vi "FinalLabview.vi"() -> ()   [LabVIEW 2021]
panel:
  out "ballcolor5":dbl
  out "ballcolor4":dbl
  out "ballcolor3":dbl
  out "ballcolor2":dbl
  out "ballcolor1":dbl
  out "DummyIndicator 5":dbl
  out "Ball Color":dbl
  out "DummyIndicator 3":dbl
  out "Ball Count":dbl
  out "Ball Color 5":string
  out "Ball Color 4":string
  out "Ball Color 3":string
  out "Ball Color 2":string
  out "Ball Color 1":string
  out "Y Coordinate 5":dbl
  out "X Coordinate 5":dbl
  out "Y Coordinate 4":dbl
  out "X Coordinate 4":dbl
  out "Y Coordinate 3":dbl
  out "X Coordinate 3":dbl
  out "Y Coordinate 2":dbl
  out "X Coordinate 2":dbl
  out "Robot Location":picture
  in  "Display History":bool
  in  "Size of Rectangle":i16
  out "Y Coordinate 1":dbl
  out "X Coordinate 1":dbl
  out "Y":dbl
  out "X":dbl
  in  "SendValue8":dbl
  in  "SendValue7":dbl
  in  "SendValue6":dbl
  in  "SendValue5":dbl
  in  "SendValue4":dbl
  in  "SendValue3":dbl
  in  "SendValue2":dbl
  in  "SendValue1":dbl
  in  "Send Button":bool
  in  "Stop Button":bool
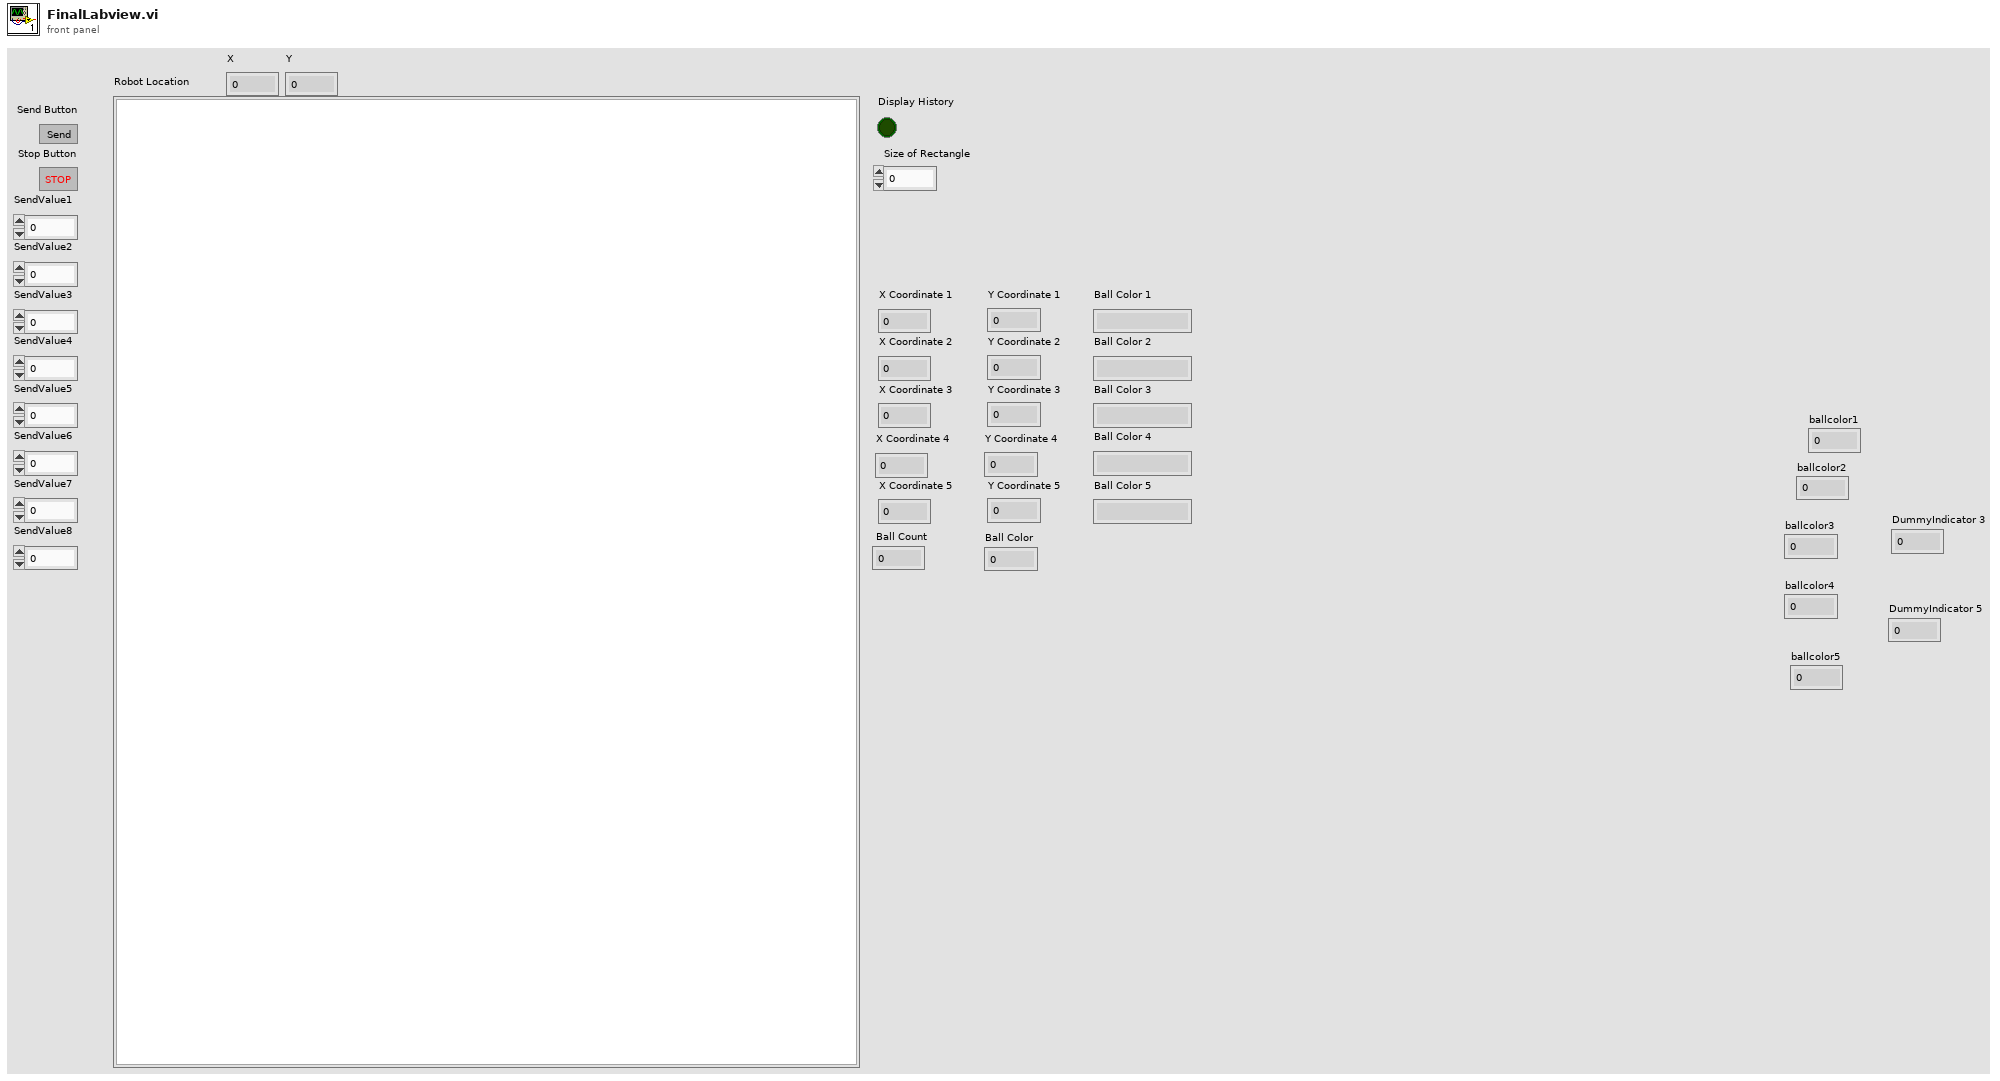
[diagram p1: front panel]
types:
  T1 = cluster{"Width":i16, "Style":enum32{"Solid", "Dash", "Dot", "DashDot", "DashDotDot"}}
  T2 = cluster{"left":i16, "top":i16, "right":i16, "bottom":i16}
  T3 = enum16{"Standard", "Buffered", "CRLF", "Immediate"}
  T4 = cluster{"Width":u16, "Style":enum32{"Solid", "Dash", "Dot", "DashDot", "DashDotDot"}}
  T5 = cluster{"default value 1":dbl, "default value 1":dbl}
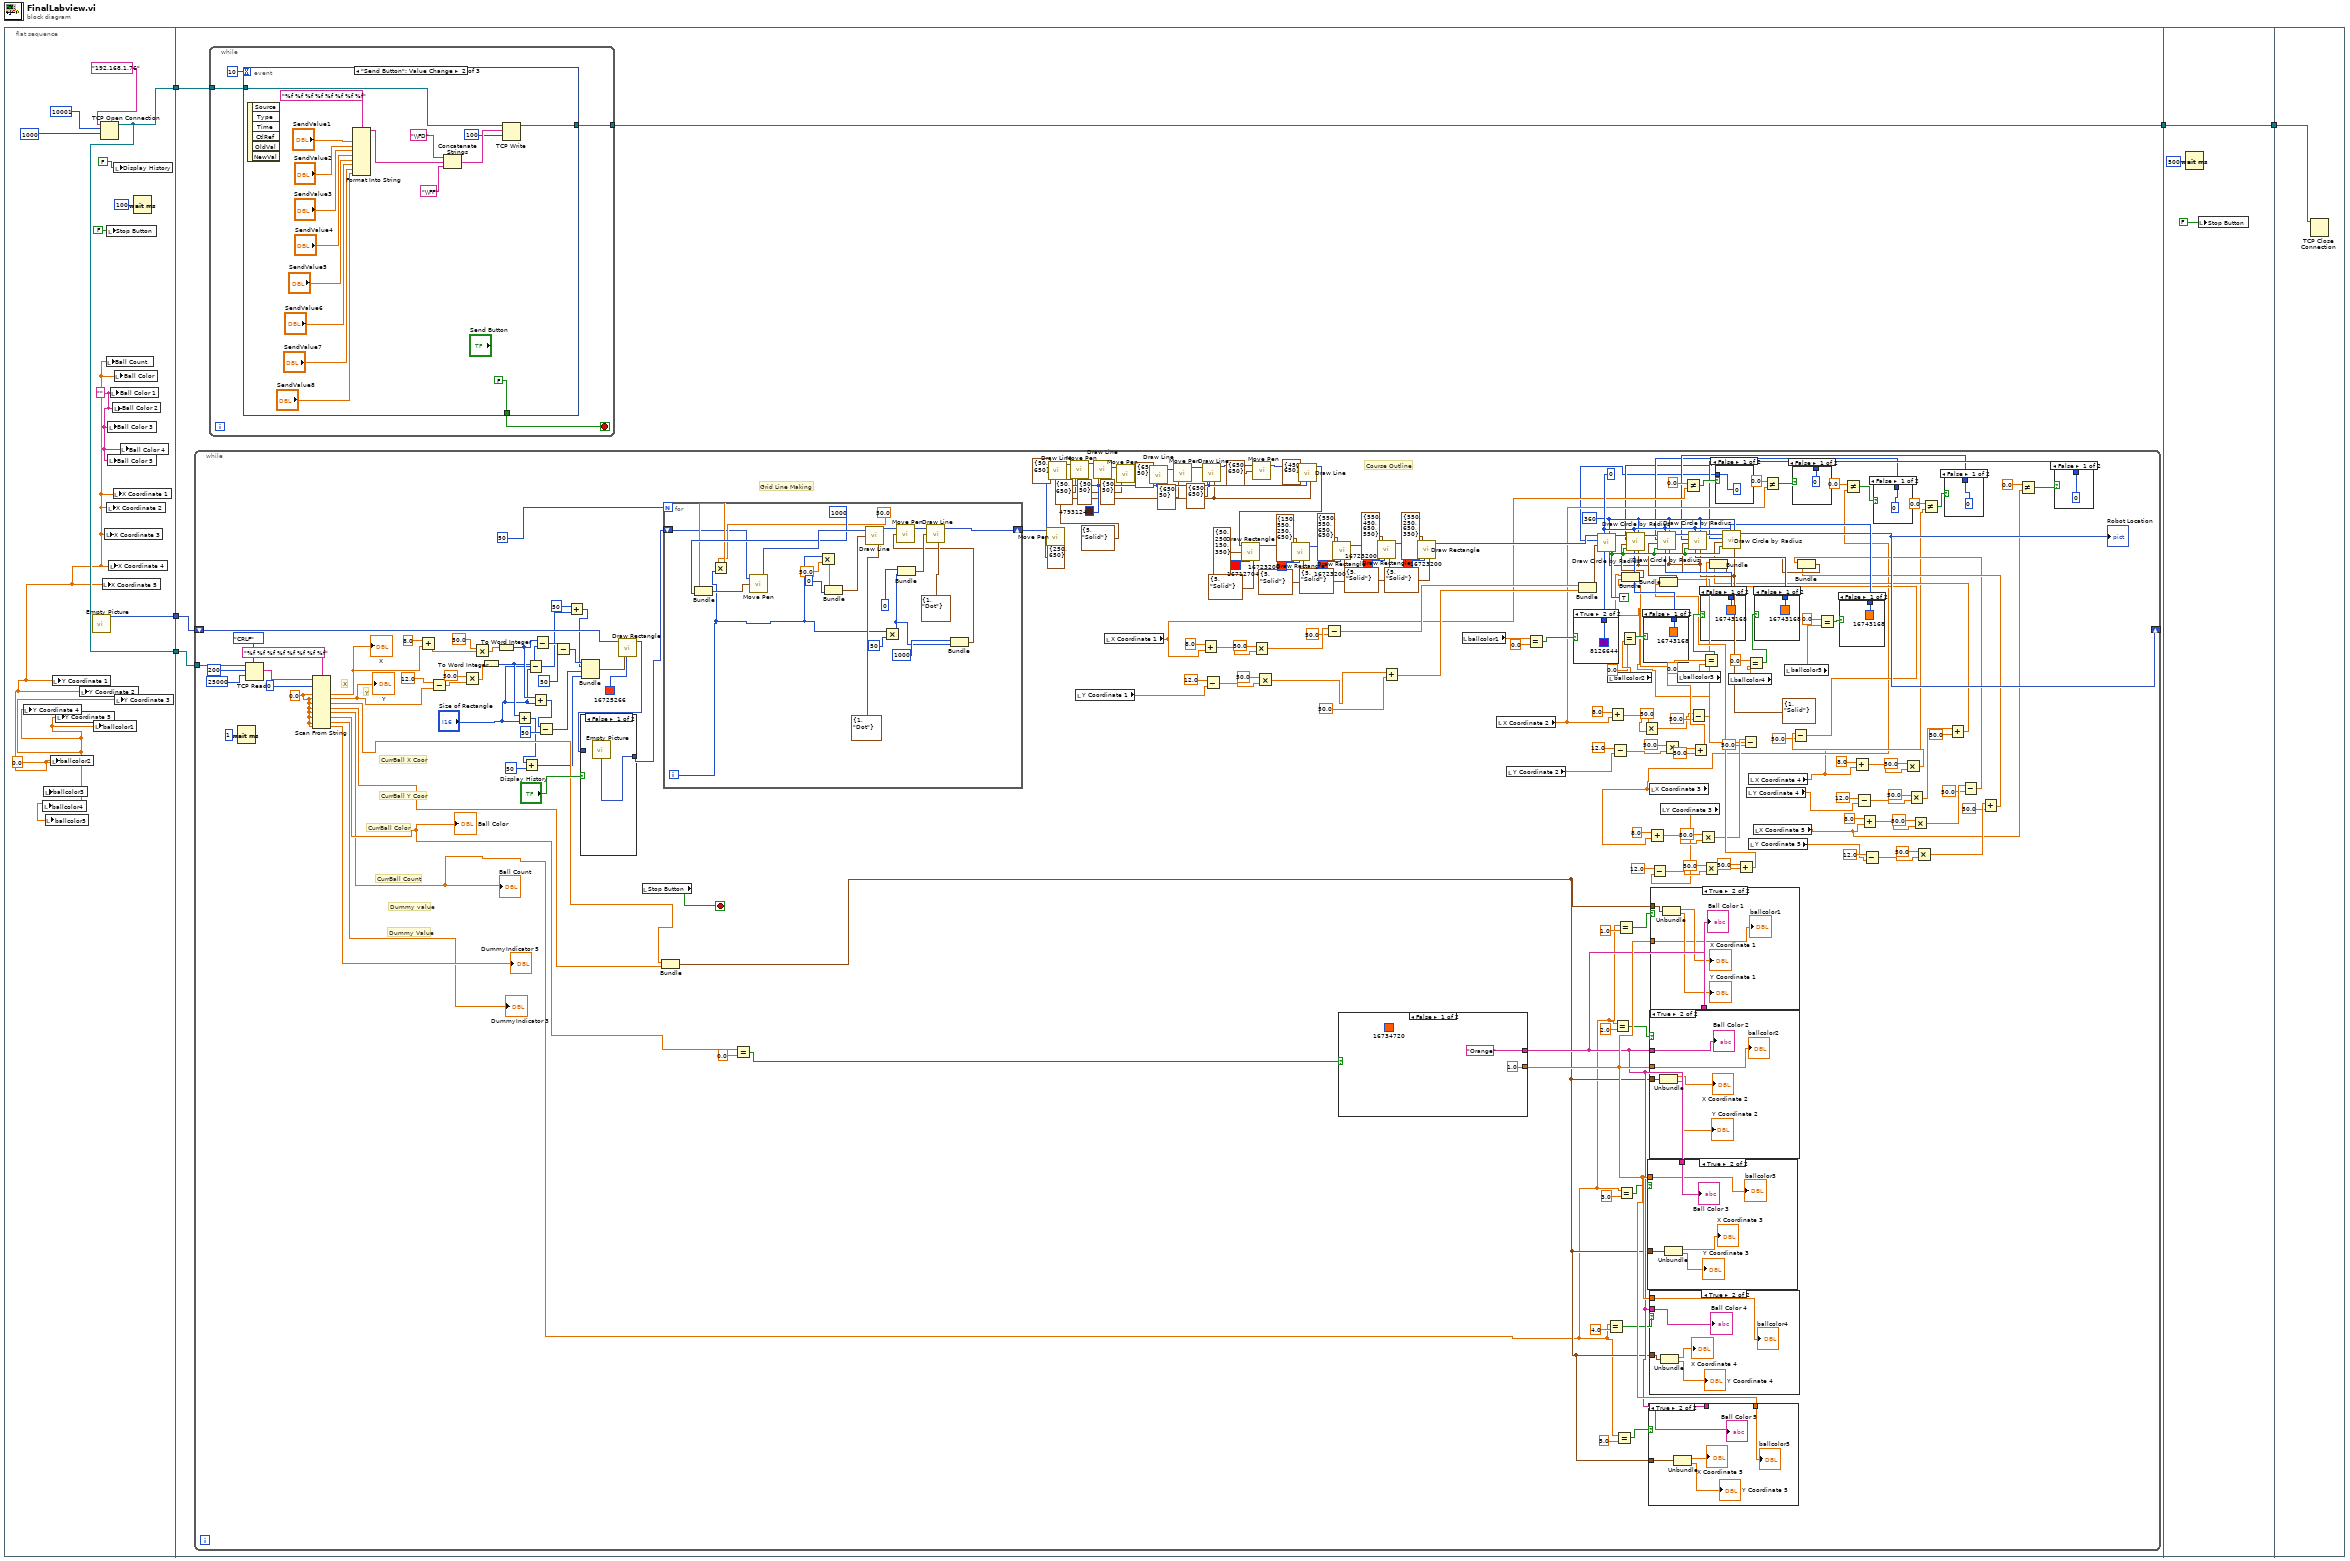
[diagram p0: block diagram]
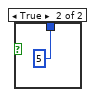
[diagram p2: hidden frame]
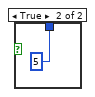
[diagram p3: hidden frame]
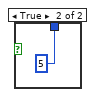
[diagram p4: hidden frame]
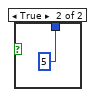
[diagram p5: hidden frame]
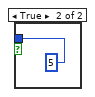
[diagram p6: hidden frame]
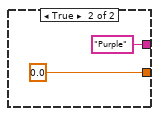
[diagram p12: hidden frame]
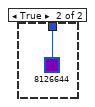
[diagram p13: hidden frame]
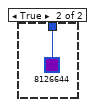
[diagram p14: hidden frame]
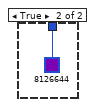
[diagram p15: hidden frame]
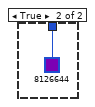
[diagram p16: hidden frame]
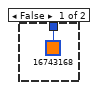
[diagram p17: hidden frame]
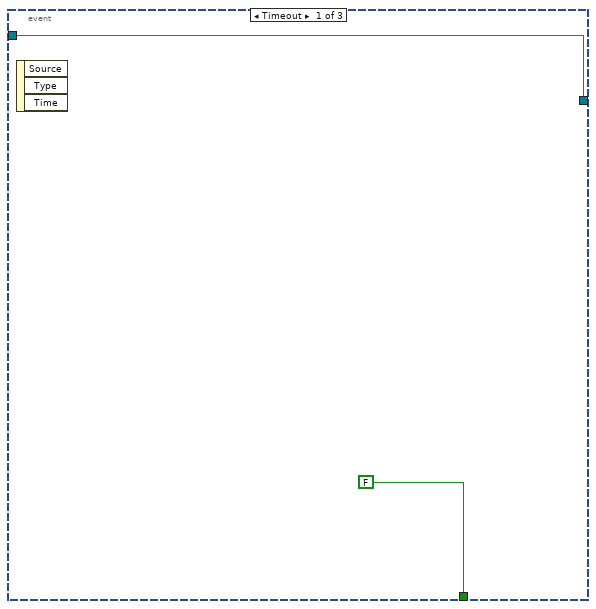
[diagram p19: hidden frame]
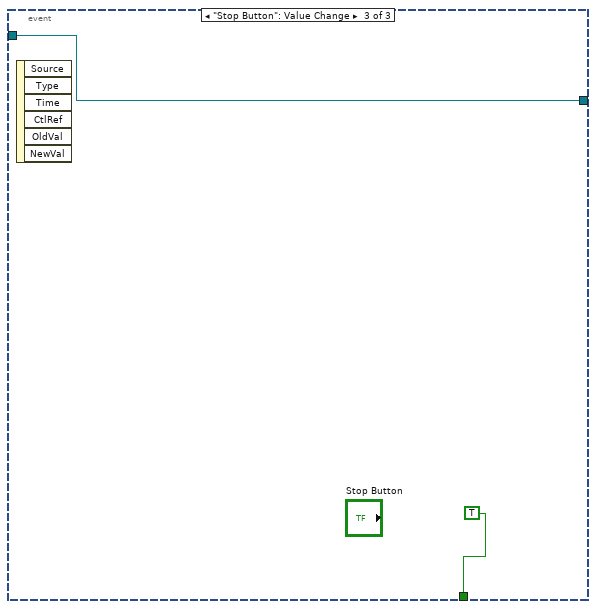
[diagram p20: hidden frame]
diagram:
  n1 = flat-sequence {
    tunnel: [w8] -> w5
    tunnel: [w10] -> w2
    tunnel: [w8] -> w1
    tunnel: w5 -> [w19]
    tunnel: [w18] -> w3
    tunnel: w2 -> [w16]
    tunnel: w1 -> [w17]
    tunnel: [w343] -> w4
    tunnel: w3 -> [w343]
    tunnel: w4 -> [w346]
    frame #0 {
      w6 = "" ("Ball Color 1")
      w7 = 0.0 ("ballcolor2")
      n2 = local write "Y Coordinate 4"(w7) -> ()
      n3 = local write "ballcolor4"(w7) -> ()
      n4 = local write "ballcolor3"(w7) -> ()
      n5 = local write "ballcolor5"(w7) -> ()
      n6 = local write "ballcolor2"(w7) -> ()
      n7 = local write "Y Coordinate 1"(w7) -> ()
      n8 = local write "Y Coordinate 5"(w7) -> ()
      n9 = local write "Y Coordinate 2"(w7) -> ()
      n10 = call "Empty Picture"() -> ("empty picture"=w10:picture)
      n11 = local write "ballcolor1"(w7) -> ()
      n12 = TCP Open Connection(address="192.168.1.76", remote port or service name=u16 10001, timeout ms (60000)=1000) -> (connection ID=w8:refnum<k5>)  [unwired: 2 in, 1 out]
      n13 = local write "X Coordinate 5"(w7) -> ()
      n14 = local write "X Coordinate 3"(w7) -> ()
      n15 = local write "Ball Count"(w7) -> ()
      n16 = local write "Stop Button"(FALSE) -> ()
      n17 = local write "X Coordinate 2"(w7) -> ()
      n18 = local write "Ball Color 3"(w6) -> ()
      n19 = local write "Ball Color 5"(w6) -> ()
      n20 = local write "X Coordinate 4"(w7) -> ()
      n21 = local write "Ball Color 1"(w6) -> ()
      n22 = local write "Ball Color 2"(w6) -> ()
      n23 = local write "X Coordinate 1"(w7) -> ()
      n24 = local write "Display History"(FALSE) -> ()
      n25 = local write "Ball Color"(w7) -> ()
      n26 = local write "Y Coordinate 3"(w7) -> ()
      n27 = local write "Ball Color 4"(w6) -> ()
      n28 = Wait (ms)(milliseconds to wait=u32 100) -> ()  [unwired: 1 out]
    }
    frame #1 {
      n29 = while {
        tunnel: w17 -> [w243]
        shift-right: [w126] -> _
        shift-left: w16 -> [w223]
        stop <- w220 stop-if-true
        w127 = T4 {"Width"=1, "Style"=enum."Solid"} ("pen")
        w152 = TRUE ("fill?(F)")
        w151 = i16 360 ("arc size(360)")
        w153 = i16 0 ("start angle(0)")
        w194 = T4 {"Width"=5, "Style"=enum."Solid"} ("pen")
        w195 = u32 4793124 ("color(black)")
        w175 = 0.0 ("default value 1")
        # "Dummy Value"
        # "CurrBall Count"
        # "Dummy value"
        # "CurrBall Color"
        # "CurrBall Y Coor"
        # "CurrBall X Coor"
        # "Y"
        # "X"
        # "Course Outline"
        # "Grid Line Making"
        n30 = Wait (ms)(milliseconds to wait=u32 1) -> ()  [unwired: 1 out]
        n31 = TCP Read(connection ID=w243, bytes to read=200, 7:T3."CRLF" ("mode (standard)"), 9:25000 ("timeout ms (25000)")) -> (data out=w239:string)  [unwired: 1 in, 2 out]
        n32 = Scan From String(format string="%f %f %f %f %f %f %f %f", input string=w239, initial scan location=u32 0, default 1=w175, default 2=w175, default 3=w175, default 4=w175, default 5=w175, default 6=w175, default 7=w175, default 8=w175) -> (output 1=w236:dbl, output 2=w174:dbl, output 3=w197:dbl, output 4=w172:dbl, output 5=w46:dbl, output 6=w169:dbl, output 7=→"DummyIndicator 3":dbl, output 8=→"DummyIndicator 5":dbl)  [unwired: 1 in, 3 out]
        "X" <- w236
        "Y" <- w174
        "Ball Count" <- w46
        "Ball Color" <- w169
        n33 = Add(x=8.0, y=w236) -> (x+y=w233:dbl)
        n34 = Subtract(x=12.0, y=w174) -> (x-y=w231:dbl)
        n35 = Multiply(x=50.0, y=w231) -> (x*y=w228:dbl)
        n36 = Multiply(x=50.0, y=w233) -> (x*y=w229:dbl)
        n37 = To Word Integer(number=w228) -> (16bit integer=w226:i16)
        n38 = To Word Integer(number=w229) -> (16bit integer=w227:i16)
        n39 = Add(x=w226, y="Size of Rectangle") -> (x+y=w44:i16)
        n40 = Add(x=w44, y=i16 50) -> (x+y=w45:i16)
        n41 = Subtract(x=w226, y="Size of Rectangle") -> (x-y=w42:i16)
        n42 = Add(x=w227, y="Size of Rectangle") -> (x+y=w164:i16)
        n43 = Subtract(x=w227, y="Size of Rectangle") -> (x-y=w161:i16)
        n44 = Subtract(x=w164, y=i16 50) -> (x-y=w163:i16)
        n45 = Subtract(x=w161, y=i16 50) -> (x-y=w162:i16)
        n46 = Add(x=i16 50, y=w42) -> (x+y=w40:i16)
        n47 = Bundle(w162, w40, w163, w45) -> (w222:cluster{i16, i16, i16, i16})  [unwired: 1 in]
        n48 = call <vilib>:"Draw Rectangle.vi"("picture"=w223, "rect"=w222, "color(black)"=u32 16725266) -> ("new picture"=w168:picture)  [unwired: 6 in]
        n49 = case shown="False" "Display History" {
          tunnel: w168 -> [_ w317]
          tunnel: [w316 w317] -> w167
          frame False {
            n50 = call "Empty Picture"() -> ("empty picture"=w316:picture)
          }
          frame True {
          }
        }
        n51 = local read "Stop Button"() -> (w220:bool)
        n52 = Bundle("default value 1"=w197, "default value 1"=w172) -> (w112:T5)  [unwired: 1 in]
        n53 = for {
          N: 50 -> [_]
          shift-right: [w310] -> w217
          shift-left: w167 -> [w294]
          i -> [w295]
          n54 = Multiply(x=50.0, y=w295) -> (x*y=w300:dbl)
          n55 = Bundle(w300, 1000) -> (w302:cluster{dbl, i32})  [unwired: 1 in]
          n56 = call <vilib>:"Move Pen.vi"("new position"=w302, "picture"=w294) -> ("new picture"=w306:picture)  [unwired: 3 in]
          n57 = Multiply(x=w295, y=50.0) -> (x*y=w314:dbl)
          n58 = Bundle(w314, 0) -> (w312:cluster{dbl, i32})  [unwired: 1 in]
          n59 = call <vilib>:"Draw Line.vi"("picture"=w306, "end point"=w312, "pen"=T4 {"Width"=1, "Style"=enum."Dot"}) -> ("new picture"=w304:picture)  [unwired: 6 in]
          n60 = Multiply(x=w295, y=50) -> (x*y=w296:i32)
          n61 = Bundle(0, w296) -> (w308:cluster{i32, i32})  [unwired: 1 in]
          n62 = Bundle(1000, w296) -> (w298:cluster{i32, i32})  [unwired: 1 in]
          n63 = call <vilib>:"Move Pen.vi"("new position"=w298, "picture"=w304) -> ("new picture"=w305:picture)  [unwired: 3 in]
          n64 = call <vilib>:"Draw Line.vi"("picture"=w305, "end point"=w308, "pen"=T4 {"Width"=1, "Style"=enum."Dot"}) -> ("new picture"=w310:picture)  [unwired: 6 in]
        }
        n65 = Equal?(x=w169, y=0.0) -> (x = y?=w113:bool)
        n66 = call <vilib>:"Move Pen.vi"("new position"=cluster{"x":i16, "y":i16} {"x"=250, "y"=650}, "picture"=w217) -> ("new picture"=w196:picture)  [unwired: 3 in]
        n67 = call <vilib>:"Draw Line.vi"("picture"=w196, "end point"=cluster{"x":i16, "y":i16} {"x"=50, "y"=650}, "color(black)"=w195, "pen"=w194) -> ("new picture"=w192:picture)  [unwired: 5 in]
        n68 = call <vilib>:"Move Pen.vi"("new position"=cluster{"x":i16, "y":i16} {"x"=50, "y"=650}, "picture"=w192) -> ("new picture"=w191:picture)  [unwired: 3 in]
        n69 = local read "Y Coordinate 1"() -> (w105:dbl)
        n70 = call <vilib>:"Draw Line.vi"("picture"=w191, "end point"=cluster{"x":i16, "y":i16} {"x"=50, "y"=50}, "color(black)"=w195, "pen"=w194) -> ("new picture"=w184:picture)  [unwired: 5 in]
        n71 = local read "X Coordinate 1"() -> (w29:dbl)
        n72 = call <vilib>:"Move Pen.vi"("new position"=cluster{"x":i16, "y":i16} {"x"=50, "y"=50}, "picture"=w184) -> ("new picture"=w183:picture)  [unwired: 3 in]
        n73 = call <vilib>:"Draw Line.vi"("picture"=w183, "end point"=cluster{"x":i16, "y":i16} {"x"=650, "y"=50}, "color(black)"=w195, "pen"=w194) -> ("new picture"=w185:picture)  [unwired: 5 in]
        n74 = call <vilib>:"Move Pen.vi"("new position"=cluster{"x":i16, "y":i16} {"x"=650, "y"=50}, "picture"=w185) -> ("new picture"=w188:picture)  [unwired: 3 in]
        n75 = Add(x=8.0, y=w29) -> (x+y=w107:dbl)
        n76 = call <vilib>:"Draw Line.vi"("picture"=w188, "end point"=cluster{"x":i16, "y":i16} {"x"=650, "y"=650}, "color(black)"=w195, "pen"=w194) -> ("new picture"=w186:picture)  [unwired: 5 in]
        n77 = Subtract(x=12.0, y=w105) -> (x-y=w106:dbl)
        n78 = call <vilib>:"Move Pen.vi"("new position"=cluster{"x":i16, "y":i16} {"x"=650, "y"=650}, "picture"=w186) -> ("new picture"=w187:picture)  [unwired: 3 in]
        n79 = Multiply(x=50.0, y=w107) -> (x*y=w75:dbl)
        n80 = Multiply(x=50.0, y=w106) -> (x*y=w73:dbl)
        n81 = call <vilib>:"Draw Line.vi"("picture"=w187, "end point"=cluster{"x":i16, "y":i16} {"x"=450, "y"=650}, "color(black)"=w195, "pen"=w194) -> ("new picture"=w190:picture)  [unwired: 5 in]
        n82 = call <vilib>:"Draw Rectangle.vi"("picture"=w190, "rect"=T2 {"left"=50, "top"=250, "right"=150, "bottom"=350}, "color(black)"=u32 16712704, "pen"=T1 {"Width"=5, "Style"=enum."Solid"}) -> ("new picture"=w213:picture)  [unwired: 5 in]
        n83 = call <vilib>:"Draw Rectangle.vi"("picture"=w213, "rect"=T2 {"left"=150, "top"=550, "right"=250, "bottom"=650}, "color(black)"=u32 16723200, "pen"=T1 {"Width"=5, "Style"=enum."Solid"}) -> ("new picture"=w212:picture)  [unwired: 5 in]
        n84 = Subtract(x=w75, y=50.0) -> (x-y=w76:dbl)
        n85 = call <vilib>:"Draw Rectangle.vi"("picture"=w212, "rect"=T2 {"left"=550, "top"=550, "right"=650, "bottom"=650}, "color(black)"=u32 16723200, "pen"=T1 {"Width"=5, "Style"=enum."Solid"}) -> ("new picture"=w211:picture)  [unwired: 5 in]
        n86 = case shown="False" w113 {
          tunnel: ["Orange" ("Ball Color 1") "Purple" ("Ball Color 1")] -> w124
          tunnel: [1.0 ("ballcolor2") 0.0 ("ballcolor2")] -> w125
          frame False {
            (unwired) u32 16734720 ("color(black)")
          }
          frame True {
          }
        }
        n87 = call <vilib>:"Draw Rectangle.vi"("picture"=w211, "rect"=T2 {"left"=550, "top"=450, "right"=650, "bottom"=550}, "color(black)"=u32 16723200, "pen"=T1 {"Width"=5, "Style"=enum."Solid"}) -> ("new picture"=w210:picture)  [unwired: 5 in]
        n88 = Add(x=w73, y=50.0) -> (x+y=w71:dbl)
        n89 = call <vilib>:"Draw Rectangle.vi"("picture"=w210, "rect"=T2 {"left"=550, "top"=250, "right"=650, "bottom"=350}, "color(black)"=u32 16723200, "pen"=T1 {"Width"=5, "Style"=enum."Solid"}) -> ("new picture"=w159:picture)  [unwired: 5 in]
        n90 = local read "ballcolor1"() -> (w150:dbl)
        n91 = local read "X Coordinate 2"() -> (w28:dbl)
        n92 = local read "Y Coordinate 2"() -> (w80:dbl)
        n93 = Equal?(x=w150, y=0.0) -> (x = y?=w148:bool)
        n94 = case shown="True" w148 {
          tunnel: [u32 16743168 ("color(black)") u32 8126644 ("color(black)")] -> w154
          frame False {
          }
          frame True {
          }
        }
        n95 = Bundle(w76, w71) -> (w160:cluster{dbl, dbl})  [unwired: 1 in]
        n96 = Equal?(x=w46, y=4.0) -> (x = y?=w120:bool)
        n97 = local read "ballcolor2"() -> (w140:dbl)
        n98 = Add(x=8.0, y=w28) -> (x+y=w100:dbl)
        n99 = Subtract(x=12.0, y=w80) -> (x-y=w99:dbl)
        n100 = Equal?(x=w46, y=2.0) -> (x = y?=w123:bool)
        n101 = Equal?(x=w46, y=5.0) -> (x = y?=w121:bool)
        n102 = Equal?(x=w46, y=1.0) -> (x = y?=w119:bool)
        n103 = Equal?(x=w46, y=3.0) -> (x = y?=w122:bool)
        n104 = Equal?(x=0.0, y=w140) -> (x = y?=w141:bool)
        n105 = Multiply(x=50.0, y=w100) -> (x*y=w48:dbl)
        n106 = case shown="False" w141 {
          tunnel: [u32 16743168 ("color(black)") u32 8126644 ("color(black)")] -> w135
          frame False {
          }
          frame True {
          }
        }
        n107 = case shown="True" w122 {
          tunnel: w124 -> [_ w269]
          tunnel: w112 -> [_ w268]
          tunnel: w125 -> [_ w265]
          frame False {
          }
          frame True {
            n108 = Unbundle(w268) -> ("default value 1"=→"X Coordinate 3":dbl, "default value 1"=→"Y Coordinate 3":dbl)
            "Ball Color 3" <- w269
            "ballcolor3" <- w265
          }
        }
        n109 = case shown="True" w121 {
          tunnel: w124 -> [_ w259]
          tunnel: w112 -> [_ w258]
          tunnel: w125 -> [_ w255]
          frame False {
          }
          frame True {
            n110 = Unbundle(w258) -> ("default value 1"=→"X Coordinate 5":dbl, "default value 1"=→"Y Coordinate 5":dbl)
            "Ball Color 5" <- w259
            "ballcolor5" <- w255
          }
        }
        n111 = local read "X Coordinate 3"() -> (w27:dbl)
        n112 = Add(x=8.0, y=w27) -> (x+y=w94:dbl)
        n113 = case shown="True" w123 {
          tunnel: w124 -> [_ w274]
          tunnel: w112 -> [_ w273]
          tunnel: w125 -> [_ w270]
          frame False {
          }
          frame True {
            n114 = Unbundle(w273) -> ("default value 1"=→"X Coordinate 2":dbl, "default value 1"=→"Y Coordinate 2":dbl)
            "Ball Color 2" <- w274
            "ballcolor2" <- w270
          }
        }
        n115 = case shown="True" w120 {
          tunnel: w124 -> [_ w264]
          tunnel: w112 -> [_ w263]
          tunnel: w125 -> [_ w260]
          frame False {
          }
          frame True {
            n116 = Unbundle(w263) -> ("default value 1"=→"X Coordinate 4":dbl, "default value 1"=→"Y Coordinate 4":dbl)
            "Ball Color 4" <- w264
            "ballcolor4" <- w260
          }
        }
        n117 = case shown="True" w119 {
          tunnel: w112 -> [_ w279]
          tunnel: w124 -> [_ w278]
          tunnel: w125 -> [_ w275]
          frame False {
          }
          frame True {
            n118 = Unbundle(w279) -> ("default value 1"=→"X Coordinate 1":dbl, "default value 1"=→"Y Coordinate 1":dbl)
            "Ball Color 1" <- w278
            "ballcolor1" <- w275
          }
        }
        n119 = local read "Y Coordinate 3"() -> (w79:dbl)
        n120 = Subtract(x=12.0, y=w79) -> (x-y=w93:dbl)
        n121 = Multiply(x=50.0, y=w99) -> (x*y=w52:dbl)
        n122 = local read "ballcolor3"() -> (w137:dbl)
        n123 = Not Equal?(x=0.0, y=w29) -> (x != y?=w35:bool)
        n124 = Subtract(x=w48, y=50.0) -> (x-y=w47:dbl)
        n125 = Add(x=w52, y=50.0) -> (x+y=w50:dbl)
        n126 = Bundle(w47, w50) -> (w131:cluster{dbl, dbl})  [unwired: 1 in]
        n127 = Multiply(x=50.0, y=w94) -> (x*y=w55:dbl)
        n128 = Equal?(x=0.0, y=w137) -> (x = y?=w136:bool)
        n129 = case shown="False" w136 {
          tunnel: [u32 16743168 ("color(black)") u32 8126644 ("color(black)")] -> w134
          frame False {
          }
          frame True {
          }
        }
        n130 = Multiply(x=50.0, y=w93) -> (x*y=w58:dbl)
        n131 = case shown="False" w35 {
          tunnel: [i16 0 ("radius") i16 5 ("radius")] -> w20
          frame False {
          }
          frame True {
          }
        }
        n132 = call <vilib>:"Draw Circle by Radius.vi"("pen"=w127, "arc size(360)"=w151, "color(black)"=w154, "start angle(0)"=w153, "fill?(F)"=w152, "pixel center"=w160, "radius"=w20, "picture"=w159) -> ("new picture"=w158:picture)  [unwired: 3 in]
        n133 = local read "ballcolor4"() -> (w143:dbl)
        n134 = Add(x=50.0, y=w58) -> (x+y=w56:dbl)
        n135 = Subtract(x=w55, y=50.0) -> (x-y=w53:dbl)
        n136 = Bundle(w53, w56) -> (w130:cluster{dbl, dbl})  [unwired: 1 in]
        n137 = Equal?(x=0.0, y=w143) -> (x = y?=w144:bool)
        n138 = local read "Y Coordinate 4"() -> (w78:dbl)
        n139 = local read "X Coordinate 4"() -> (w26:dbl)
        n140 = local read "Y Coordinate 5"() -> (w77:dbl)
        n141 = local read "X Coordinate 5"() -> (w25:dbl)
        n142 = case shown="False" w144 {
          tunnel: [u32 16743168 ("color(black)") u32 8126644 ("color(black)")] -> w133
          frame False {
          }
          frame True {
          }
        }
        n143 = Not Equal?(x=0.0, y=w28) -> (x != y?=w36:bool)
        n144 = local read "ballcolor5"() -> (w146:dbl)
        n145 = case shown="False" w36 {
          tunnel: [i16 0 ("radius") i16 5 ("radius")] -> w21
          frame False {
          }
          frame True {
          }
        }
        n146 = call <vilib>:"Draw Circle by Radius.vi"("pen"=w127, "arc size(360)"=w151, "color(black)"=w135, "start angle(0)"=w153, "fill?(F)"=w152, "pixel center"=w131, "radius"=w21, "picture"=w158) -> ("new picture"=w157:picture)  [unwired: 3 in]
        n147 = Equal?(x=0.0, y=w146) -> (x = y?=w147:bool)
        n148 = case shown="False" w147 {
          tunnel: [u32 16743168 ("color(black)") u32 8126644 ("color(black)")] -> w132
          frame False {
          }
          frame True {
          }
        }
        n149 = Not Equal?(x=0.0, y=w27) -> (x != y?=w37:bool)
        n150 = Add(x=8.0, y=w26) -> (x+y=w88:dbl)
        n151 = Subtract(x=12.0, y=w78) -> (x-y=w87:dbl)
        n152 = Add(x=8.0, y=w25) -> (x+y=w82:dbl)
        n153 = Subtract(x=12.0, y=w77) -> (x-y=w81:dbl)
        n154 = case shown="False" w37 {
          tunnel: [i16 0 ("radius") i16 5 ("radius")] -> w22
          frame False {
          }
          frame True {
          }
        }
        n155 = call <vilib>:"Draw Circle by Radius.vi"("pen"=w127, "arc size(360)"=w151, "color(black)"=w134, "start angle(0)"=w153, "fill?(F)"=w152, "pixel center"=w130, "radius"=w22, "picture"=w157) -> ("new picture"=w156:picture)  [unwired: 3 in]
        n156 = Multiply(x=50.0, y=w88) -> (x*y=w64:dbl)
        n157 = Subtract(x=w64, y=50.0) -> (x-y=w62:dbl)
        n158 = Multiply(x=50.0, y=w87) -> (x*y=w61:dbl)
        n159 = Multiply(x=50.0, y=w82) -> (x*y=w67:dbl)
        n160 = Multiply(x=50.0, y=w81) -> (x*y=w69:dbl)
        n161 = Not Equal?(x=0.0, y=w26) -> (x != y?=w38:bool)
        n162 = case shown="False" w38 {
          tunnel: [i16 0 ("radius") i16 5 ("radius")] -> w23
          frame False {
          }
          frame True {
          }
        }
        n163 = Add(x=w61, y=50.0) -> (x+y=w59:dbl)
        n164 = Bundle(w62, w59) -> (w129:cluster{dbl, dbl})  [unwired: 1 in]
        n165 = call <vilib>:"Draw Circle by Radius.vi"("pen"=w127, "arc size(360)"=w151, "color(black)"=w133, "start angle(0)"=w153, "fill?(F)"=w152, "pixel center"=w129, "radius"=w23, "picture"=w156) -> ("new picture"=w155:picture)  [unwired: 3 in]
        n166 = Subtract(x=w67, y=50.0) -> (x-y=w65:dbl)
        n167 = Add(x=w69, y=50.0) -> (x+y=w70:dbl)
        n168 = Bundle(w65, w70) -> (w128:cluster{dbl, dbl})  [unwired: 1 in]
        n169 = Not Equal?(x=0.0, y=w25) -> (x != y?=w39:bool)
        n170 = case shown="False" w39 {
          tunnel: [i16 0 ("radius") i16 5 ("radius")] -> w24
          frame False {
          }
          frame True {
          }
        }
        n171 = call <vilib>:"Draw Circle by Radius.vi"("pen"=w127, "arc size(360)"=w151, "color(black)"=w132, "start angle(0)"=w153, "fill?(F)"=w152, "pixel center"=w128, "radius"=w24, "picture"=w155) -> ("new picture"=w126:picture)  [unwired: 3 in]
        "Robot Location" <- w126
      }
      n172 = while {
        tunnel: w19 -> [w319]
        tunnel: [w318] -> w18
        stop <- w320 stop-if-true
        n173 = event shown="[1] \"Send Button\": Value Change" {
          selector: _ -> [_ _ _]
          dyn-events: _ -> [_ _ _]
          timeout: 10 -> [_ _ _]
          tunnel: [FALSE FALSE TRUE] -> w320
          tunnel: w319 -> [w322 w325 w341]
          tunnel: [w322 w324 w341] -> w318
          event Timeout {
            n174 = event-data() -> ()  [unwired: 1 in, 3 out]
          }
          event "Send Button": Value Change {
            n175 = event-data() -> ()  [unwired: 1 in, 6 out]
            n176 = Format Into String(format string="%f %f %f %f %f %f %f %f", "SendValue1", "SendValue2", "SendValue3", "SendValue4", "SendValue5", "SendValue6", "SendValue7", "SendValue8") -> (resulting string=w327:string)  [unwired: 2 in, 1 out]
            n177 = Concatenate Strings("\\FD" ("string"), w327, "\\FF" ("string")) -> (w330:string)
            n178 = TCP Write(connection ID=w325, data in=w330, 9:100 ("timeout ms (25000)")) -> (connection ID out=w324:refnum<k5>)  [unwired: 1 in, 2 out]
          }
          event "Stop Button": Value Change {
            n179 = event-data() -> ()  [unwired: 1 in, 6 out]
          }
        }
      }
    }
    frame #2 {
      n180 = Wait (ms)(milliseconds to wait=u32 500) -> ()  [unwired: 1 out]
      n181 = local write "Stop Button"(FALSE) -> ()
    }
    frame #3 {
      n182 = TCP Close Connection(connection ID=w346) -> ()  [unwired: 2 in, 2 out]
    }
  }
